vi "Write Function (0_ DC Voltage).vi"(8 "error in (no error)":errorcluster, 10 "Function (0: DC Voltage)":T1=1 items=["DC Volts"=1, "AC Volts"=2, "DC Current"=3, "AC Current"=4, "2 Wire Resistance"=5, "4 Wire Resistance"=101, "AC + DC Volts"=106, "AC + DC Current"=107, "Frequency"=104, "Period"=105, "AC Volts (Random Sampling)"=1001, "AC Volts (Sync Sampling)"=1002, "AC + DC Volts (Random Sampling)"=1003, "AC + DC Volts (Sync Sampling)"=1004, "AC Couple (Direct-Sampling)"=1005, "DC Couple (Direct-Sampling)"=1006, "AC Couple (Sub-Sampling)"=1007, "DC Couple (Sub-Sampling)"=1008], 11 "Agilent_3458 in":refnum<class "Agilent_3458.lvclass">) -> (0 "error out":errorcluster, 3 "Agilent_3458 out":refnum<class "Agilent_3458.lvclass">)   [LabVIEW 2018, in "DigitizerPlugins.lvlib" / "Agilent_3458.lvclass"]
uses:
  Agilent_3458.lvclass
  Typedefs/MeasurementFunction.ctl
  Agilent_3458.lvclass/Agilent_3458.ctl
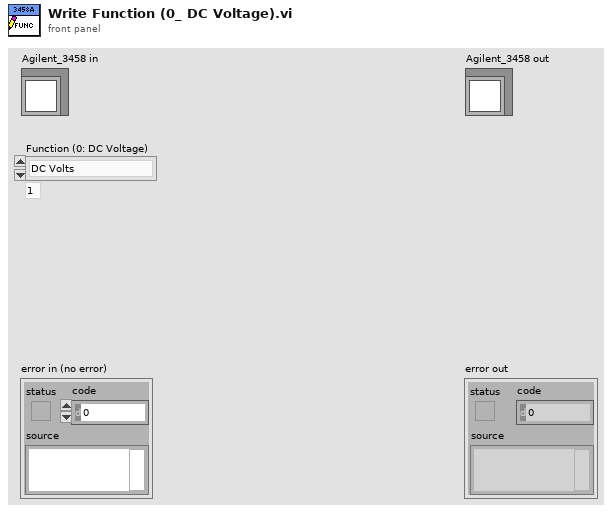
[diagram p1: front panel]
types:
  T1 = typedef "DigitizerPlugins.lvlib/Agilent_3458.lvclass/MeasurementFunction.ctl" = i32
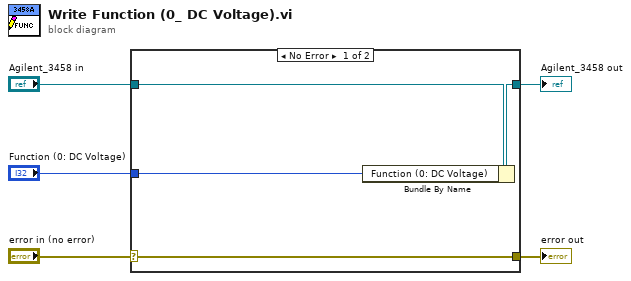
[diagram p0: block diagram]
diagram:
  n1 = case shown="No Error" "error in (no error)" {
    selector: "error in (no error)" -> [w9 w10]
    tunnel: [w9 w10] -> w4
    tunnel: [w7 w11] -> w2
    tunnel: "Agilent_3458 in" -> [w8 w11]
    tunnel: "Function (0: DC Voltage)" -> [w6 _]
    frame No Error {
      n2 = Bundle By Name(cluster=w8, "Function (0: DC Voltage)"=w6) -> (w7:refnum<class "Agilent_3458.lvclass">)
    }
    frame Error {
    }
  }
  "error out" <- w4
  "Agilent_3458 out" <- w2
